vi "Load Properties from Configuration File.vi"(6 "String Properties":string[](array[string]), 7 "Section":string, 8 "error in":errorcluster, 9 "Boolean Properties":string[](array[string]), 10 "Numeric Properties":string[](array[string]), 11 "Item Reference In":T1 format="%.0x") -> (0 "error out":errorcluster, 3 "Item Device Reference Out":T1 format="%.0x")   [LabVIEW 2018, in "Embedded Data Logger System Explorer.lvlib"]
uses:
  Embedded Data Logger System Explorer.lvlib
  <vilib>/NI Veristand/Custom Device API/Custom Device Item Ref.ctl
  <vilib>/Utility/config.llb/Read Key (String).vi
  <vilib>/NI Veristand/Custom Device API/Set Item Property (String).vi
  <vilib>/Utility/config.llb/Read Key (Double).vi
  <vilib>/NI Veristand/Custom Device API/Set Item Property (Double).vi
  <vilib>/Utility/config.llb/Read Key (Boolean).vi
  <vilib>/NI Veristand/Custom Device API/Set Item Property (Boolean).vi
  <vilib>/Utility/config.llb/NI_LVConfig.lvlib
  <vilib>/NI Veristand/Custom Device API/Custom Device API.lvlib
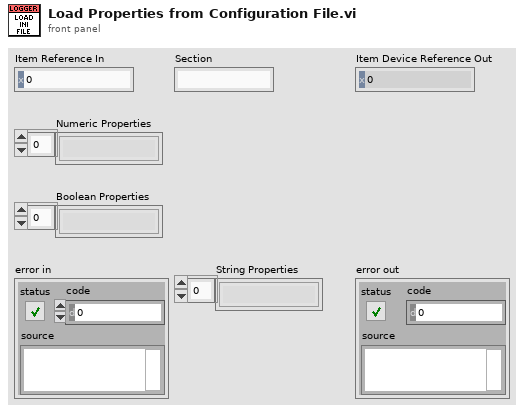
[diagram p1: front panel]
types:
  T1 = typedef "Custom Device API.lvlib/Custom Device Item Ref.ctl" = u64
  T2 = typedef "NI_LVConfig.lvlib/Config Data RefNum.ctl" = refnum<k1>
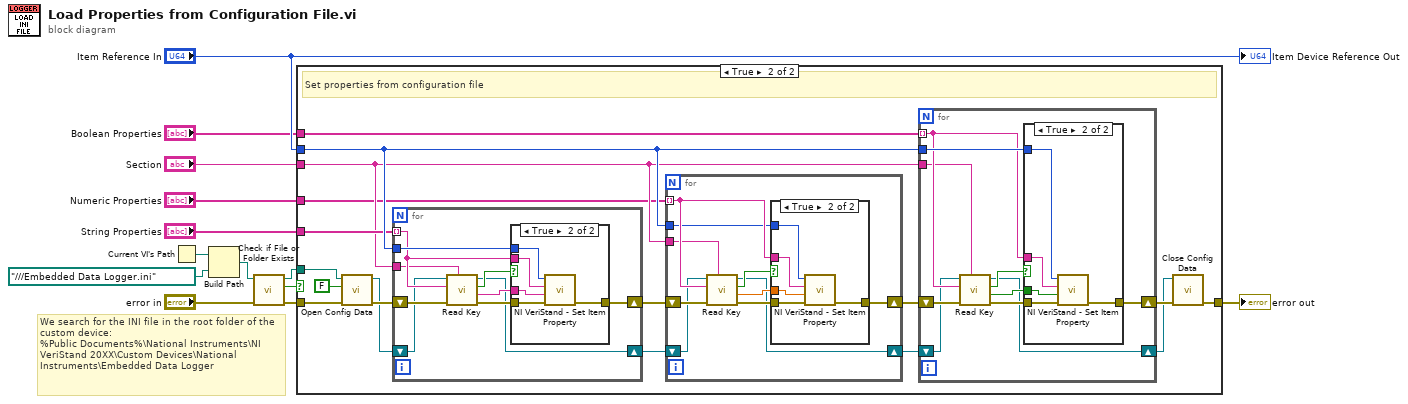
[diagram p0: block diagram]
diagram:
  # "We search for the INI file in the root folder of the custom device:\n%Public Documents%\\National Instruments\\NI VeriStand 20XX\\Custom Devices\\National Instruments\\Embedded Data Logger"
  n1 = Current VI's Path() -> (path=w7:path)
  n2 = Build Path(base path=w7, name or relative path=path "../../../Embedded Data Logger.ini") -> (appended path=w6:path)
  n3 = call <vilib>:"Check if File or Folder Exists.vi"("error in (no error)"="error in", "path"=w6) -> ("error out"=w13:errorcluster, "file or folder exists?"=w12:bool, "dup path"=w11:path)  [unwired: 7 in]
  n4 = case shown="True" w12 {
    tunnel: w13 -> [w14 w31]
    tunnel: w11 -> [_ w30]
    tunnel: [w14 w29] -> w9
    tunnel: "Item Reference In" -> [_ w23]
    tunnel: "String Properties" -> [_ w18]
    tunnel: "Section" -> [_ w17]
    tunnel: "Numeric Properties" -> [_ w16]
    tunnel: "Boolean Properties" -> [_ w15]
    frame False {
      # "If there's no configuration file, do nothing"
    }
    frame True {
      # "Set properties from configuration file"
      n5 = call <vilib>:"Open Config Data.vi"("error in (no error)"=w31, "create file if necessary (T)"=FALSE, "configuration file path"=w30) -> ("error out"=w27:errorcluster, "refnum"=w22:T2)  [unwired: 6 in, 1 out]
      n6 = for {
        shift-right: [w40] -> w26
        shift-left: w27 -> [w41]
        tunnel: w18 -> [w35] mode=indexing
        tunnel: w23 -> [w36]
        shift-right: [w33] -> w21
        shift-left: w22 -> [w34]
        tunnel: w17 -> [w32]
        n7 = call-poly <vilib>:"Read Key.vi"("section"=w32, "error in (no error)"=w41, "key"=w35, "refnum"=w34) -> ("error out"=w39:errorcluster, "value"=w37:string, "found?"=w38:bool, "refnum out"=w33:T2)  [unwired: 4 in]
        n8 = case shown="True" w38 {
          tunnel: w39 -> [w42 w47]
          tunnel: [w42 w46] -> w40
          tunnel: w37 -> [_ w45]
          tunnel: w36 -> [_ w44]
          tunnel: w35 -> [_ w43]
          frame False {
          }
          frame True {
            n9 = call-poly <vilib>:"NI VeriStand - Set Item Property.vi"("error in (no error)"=w47, "Value"=w45, "Property Name"=w43, "Item Ref in"=w44) -> ("error out"=w46:errorcluster)  [unwired: 5 in, 2 out]
          }
        }
      }
      n10 = for {
        shift-right: [w72] -> w25
        shift-left: w26 -> [w73]
        tunnel: w16 -> [w68] mode=indexing
        tunnel: w23 -> [w67]
        shift-right: [w65] -> w20
        shift-left: w21 -> [w66]
        tunnel: w17 -> [w64]
        n11 = call-poly <vilib>:"Read Key.vi"("section"=w64, "error in (no error)"=w73, "key"=w68, "refnum"=w66) -> ("error out"=w71:errorcluster, "value"=w69:dbl, "found?"=w70:bool, "refnum out"=w65:T2)  [unwired: 4 in]
        n12 = case shown="True" w70 {
          tunnel: w71 -> [w74 w79]
          tunnel: [w74 w78] -> w72
          tunnel: w69 -> [_ w77]
          tunnel: w68 -> [_ w76]
          tunnel: w67 -> [_ w75]
          frame False {
          }
          frame True {
            n13 = call-poly <vilib>:"NI VeriStand - Set Item Property.vi"("error in (no error)"=w79, "Value"=w77, "Property Name"=w76, "Item Ref in"=w75) -> ("error out"=w78:errorcluster)  [unwired: 5 in, 2 out]
          }
        }
      }
      n14 = for {
        shift-right: [w56] -> w24
        shift-left: w25 -> [w57]
        tunnel: w15 -> [w51] mode=indexing
        tunnel: w23 -> [w52]
        shift-right: [w49] -> w19
        shift-left: w20 -> [w50]
        tunnel: w17 -> [w48]
        n15 = call-poly <vilib>:"Read Key.vi"("section"=w48, "error in (no error)"=w57, "key"=w51, "refnum"=w50) -> ("error out"=w55:errorcluster, "value"=w53:bool, "found?"=w54:bool, "refnum out"=w49:T2)  [unwired: 4 in]
        n16 = case shown="True" w54 {
          tunnel: w55 -> [w58 w63]
          tunnel: [w58 w62] -> w56
          tunnel: w53 -> [_ w61]
          tunnel: w52 -> [_ w59]
          tunnel: w51 -> [_ w60]
          frame False {
          }
          frame True {
            n17 = call-poly <vilib>:"NI VeriStand - Set Item Property.vi"("error in (no error)"=w63, "Value"=w61, "Property Name"=w60, "Item Ref in"=w59) -> ("error out"=w62:errorcluster)  [unwired: 5 in, 2 out]
          }
        }
      }
      n18 = call <vilib>:"Close Config Data.vi"("error in (no error)"=w24, "refnum"=w19) -> ("error out"=w29:errorcluster)  [unwired: 8 in, 1 out]
    }
  }
  "error out" <- w9
  "Item Device Reference Out" <- "Item Reference In"
